vi "InitSessionCV.vi"() -> (1 "session out":refnum<k35>, 4 "error out":errorcluster)   [LabVIEW 2018]
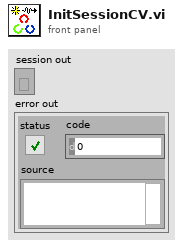
[diagram p1: front panel]
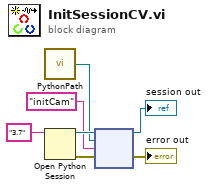
[diagram p0: block diagram]
diagram:
  n1 = call "PythonPath.vi"() -> ("path to .py"=w1:path)
  n2 = Open Python Session(python version="3.7" ("Python version")) -> (session out=w4:refnum<k35>, error out=w3:errorcluster)  [unwired: 2 in]
  n3 = node(w4, w1, "initCam" ("function name"), w3) -> (→"session out":refnum<k35>, →"error out":errorcluster)  [unwired: 2 in, 2 out]
